vi "GetHostControlStatus.vi"(8 "error in (no error)":errorcluster, 11 "SM1000-control in":T1) -> (0 "error out":errorcluster, 1 "Host in control?":bool, 3 "SM1000-control out":T1)   [LabVIEW 2013, in "HardwareCharacterization.lvlib" / "HC-SM1000.lvclass"]
doc: "Returns the current EC1000 control status of this remote control session.\n\n\"4\": Control has been granted to this session.\n\"5\": This session is not in exclusive control of the EC1000.\n\nCommand: \"GetHostControlStatus\" or 4\nReturns: \"4\"/\"5\""
uses:
  HC-SM1000.lvclass
  Object-reference.ctl
  HC-SM1000.lvclass/HC-SM1000.ctl
  Custom-errors.ctl
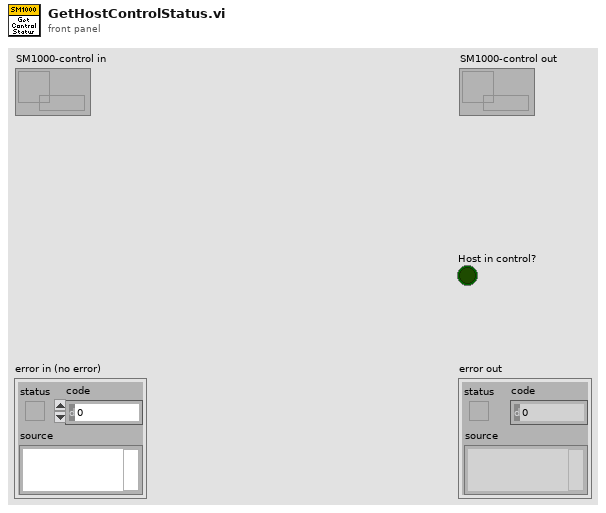
[diagram p1: front panel]
types:
  T1 = typedef "HardwareCharacterization.lvlib/HC-SM1000.lvclass/Object-reference.ctl" = refnum<data-value>
  T2 = typedef "HardwareCharacterization.lvlib/HC-SM1000.lvclass/Custom-errors.ctl" = enum16{"No error", "Not implemented", "Command not recognized", "Invalid input", "No connection", "Timeout", "Resource not loaded"}
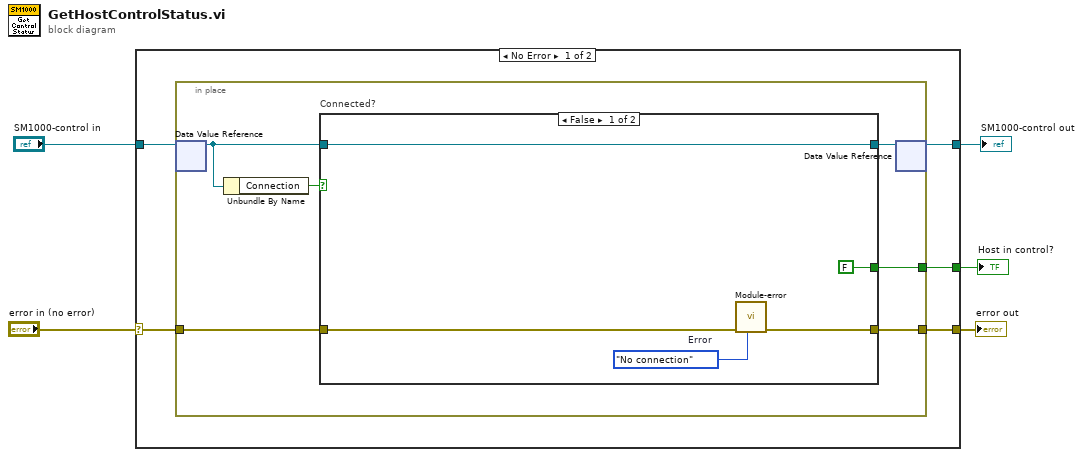
[diagram p0: block diagram]
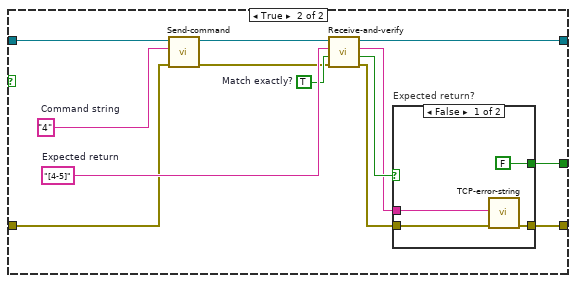
[diagram p2: hidden frame]
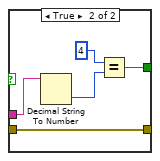
[diagram p3: hidden frame]
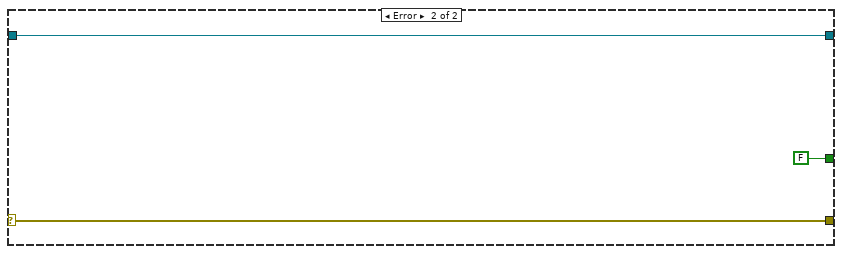
[diagram p4: hidden frame]
diagram:
  n1 = case shown="No Error" "error in (no error)" {
    selector: "error in (no error)" -> [w8 w46]
    tunnel: [w7 w46] -> w4
    tunnel: [w9 w45] -> w2
    tunnel: "SM1000-control in" -> [w10 w45]
    tunnel: [w6 FALSE] -> w1
    frame No Error {
      n2 = in-place {
        in-place-border: w8 -> [w16]
        in-place-border: [w13] -> w7
        in-place-border: [w11] -> w6
        n3 = in-place-dvr #1(w10) -> (w14:refnum<class "HC-SM1000.lvclass">)  [unwired: 1 out]
        n4 = Unbundle By Name(w14) -> ("Connection"=w15:bool)
        n5 = case "Connected?" shown="False" w15 {
          tunnel: w16 -> [w21 w26]
          tunnel: w14 -> [w19 w34]
          tunnel: [w20 w24] -> w13
          tunnel: [w19 w23] -> w12
          tunnel: [FALSE w22] -> w11
          frame False {
            w17 = Custom-errors."No connection"  # Error
            n6 = call "Module-error.vi"("Error"=w17, "error in (no error)"=w21) -> ("error out"=w20:errorcluster)  [unwired: 9 in]
          }
          frame True {
            w30 = TRUE  # Match exactly?
            w31 = "[4-5]"  # Expected return
            w32 = "4"  # Command string
            n7 = call "Send-command.vi"("error in (no error)"=w26, "Command string"=w32, "SM1000-control in"=w34) -> ("error out"=w29:errorcluster, "SM1000-control out"=w33:refnum<class "HC-SM1000.lvclass">)  [unwired: 7 in]
            n8 = call "Receive-and-verify.vi"("error in (no error)"=w29, "Match exactly?"=w30, "Expected return string"=w31, "SM1000-control in"=w33) -> ("error out"=w25:errorcluster, "Verified?"=w28:bool, "Return string"=w27:string, "SM1000-control out"=w23:refnum<class "HC-SM1000.lvclass">)  [unwired: 4 in]
            n9 = case "Expected return?" shown="False" w28 {
              tunnel: w27 -> [w38 w42]
              tunnel: w25 -> [w37 w43]
              tunnel: [w36 w43] -> w24
              tunnel: [FALSE w39] -> w22
              frame False {
                n10 = call "TCP-error-string.vi"("error in (no error)"=w37, "Retun code"=w38) -> ("error out"=w36:errorcluster)  [unwired: 9 in]
              }
              frame True {
                n11 = Decimal String To Number(string=w42) -> (number=w41:i32)  [unwired: 2 in, 1 out]
                n12 = Equal?(x=4, y=w41) -> (x = y?=w39:bool)
              }
            }
          }
        }
        n13 = in-place-dvr #1(w12) -> (w9:T1)  [unwired: 1 out]
      }
    }
    frame Error {
    }
  }
  "error out" <- w4
  "SM1000-control out" <- w2
  "Host in control?" <- w1
